vi "Unregister.vi"(8 "Error In":errorcluster, 10 "Listener ID":string, 11 "Listeners In":refnum<queue>[](array[refnum])) -> (0 "Error Out":errorcluster, 3 "Listeners Out":refnum<queue>[](array[refnum]))   [LabVIEW 2025, in "LOGlib_LV2025.lvlib"]
uses:
  LOGlib_LV2025.lvlib
  Type Definitions/Statement.ctl
  Type Definitions/Tag.ctl
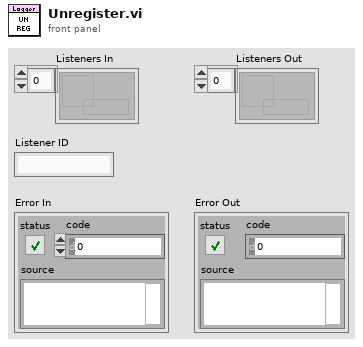
[diagram p1: front panel]
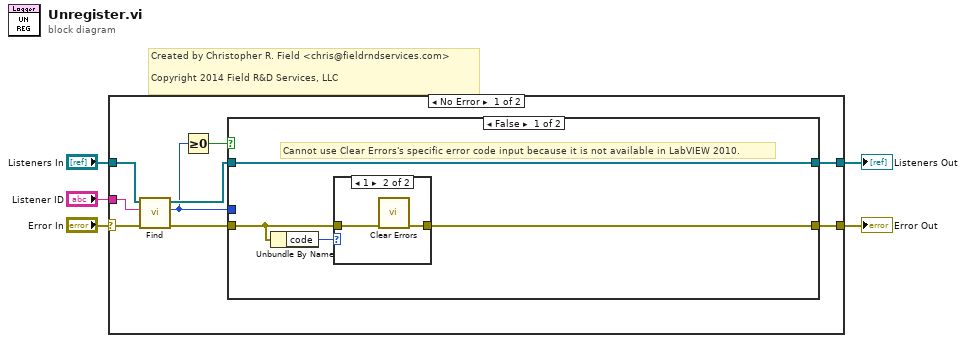
[diagram p0: block diagram]
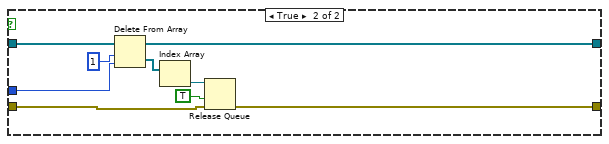
[diagram p3: hidden frame]
diagram:
  # "Created by Christopher R. Field <chris@fieldrndservices.com>\n\nCopyright 2014 Field R&D Services, LLC"
  n1 = case shown="No Error" "Error In" {
    selector: "Error In" -> [w7 w31]
    tunnel: [w14 w31] -> w5
    tunnel: [w13 w32] -> w4
    tunnel: "Listeners In" -> [w11 w32]
    tunnel: "Listener ID" -> [w8 _]
    frame No Error {
      n2 = call "Find.vi"("Error In"=w7, "Listener ID"=w8, "Listeners In"=w11) -> ("Error Out"=w6:errorcluster, "Index"=w9:i32, "Listeners Out"=w10:refnum<queue>[])  [unwired: 6 in]
      n3 = Greater Or Equal To 0?(x=w9) -> (x >= 0?=w12:bool)
      n4 = case shown="False" w12 {
        tunnel: w10 -> [w18 w30]
        tunnel: w9 -> [_ w28]
        tunnel: [w18 w27] -> w13
        tunnel: w6 -> [w16 w24]
        tunnel: [w15 w23] -> w14
        frame False {
          # "Cannot use Clear Errors's specific error code input because it is not available in LabVIEW 2010."
          n5 = Unbundle By Name(w16) -> ("code"=w17:i32)
          n6 = case shown="1" w17 {
            tunnel: w16 -> [w19 w21]
            tunnel: [w19 w20] -> w15
            frame 0, Default {
            }
            frame 1 {
              n7 = call <vilib>:"Clear Errors.vi"("error in (no error)"=w21) -> ("error out"=w20:errorcluster)  [unwired: 5 in, 1 out]
            }
          }
        }
        frame True {
          n8 = Delete From Array(array=w30, length=1, index=w28) -> (deleted portion=w26:refnum<queue>[], array with subset deleted=w27:refnum<queue>[])
          n9 = Index Array(array=w26) -> (element=w25:refnum<queue>)  [unwired: 1 in]
          n10 = Release Queue(queue=w25, force destroy? (F)=TRUE, error in (no error)=w24) -> (error out=w23:errorcluster)  [unwired: 2 out]
        }
      }
    }
    frame Error {
    }
  }
  "Error Out" <- w5
  "Listeners Out" <- w4
